vi "ProcessData(SubVI).vi"(5 "Queue":refnum<queue>) -> ()   [LabVIEW 2013, in "main.lvlib"]
uses:
  main.lvlib
  Controls/Enum Variables.ctl
  Controls/Enum User Events.ctl
  Controls/Enum Globals.ctl
  Controls/Enum Process Data.ctl
  CreatePDF.vi
panel:
  out "Blue":dbl[][](graph)
  out "Blue index":dbl format="%d%%"
  in  "ResetBlueBtn":bool
  in  "ZoomBlueBtn":bool
  out "Blue Pressure":dbl
  out "Red":dbl[][](graph)
  out "Armpressure":dbl
  in  "System Stop Button":bool
  in  "GraphSelection(Red:F)":bool
  in  "Cursor Mode":bool
  in  "ResetFrontImage":bool
  out "Red index":dbl format="%d%%"
  out "Red Pressure":dbl
  in  "ResetRedBtn":bool
  in  "ZoomRedBtn":bool
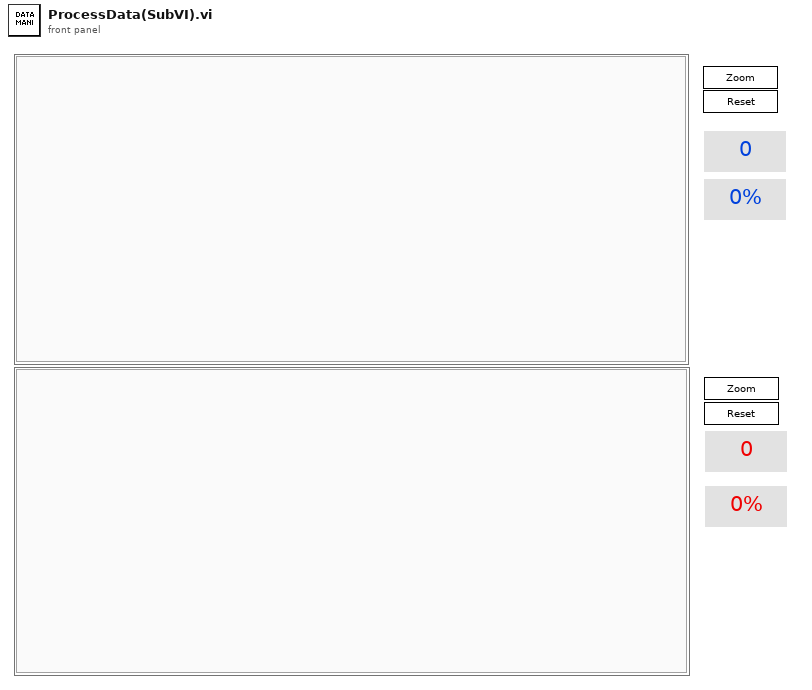
[diagram p1: front panel]
types:
  T1 = typedef "main.lvlib/Enum Process Data.ctl" = enum16{"Init", "Set Cursor Mode", "Set Data Path", "Get All"}
  T2 = typedef "main.lvlib/Enum Variables.ctl" = enum16{"SetAcqFilter", "GetAcqFilter", "Set Filter", "Get Filter", "Set Height", "Get Height", "Set Recorded Height", "Get Recorded Height", "Set Blue Pressure", "Get Blue Pressure", "Set Red Pressure", "Get Red Pressure", "Init", "Reset Pressure", "Set Red Cursors", "Get Red Cursors", "Set Blue Cursors", "Get Blue Cursors", "Set Language", "Get Language", "Set Active Graphs", "Get ActiveGraphs", "Set Method", "Get Method", "Set Encryption", "Get Encryption", "Set ExcelVersion", "Get ExcelVersion", "Set DICOM Avail", "Get DICOM Avail", "Set DICOM Encode", "Get DICOM Encode", "Set JournalExport", "Get JournalExport", "Set Sequence", "Get Sequence", "Set DAQ Connected", "Get DAQ Connected", "Set Current Graph", "Get Current Graph", "Set General Settings", "Get Hyphenation", "Set Arm Calc Method", "Get Arm Calc Method", "Set Dicom Tags", "Get Dicom Tags", "Set BT Serial", "Get BT Serial", "Set BT Accepted Serials", "Get BT Accepted Serials", "Get BT License", "Set BT License"}
  T3 = typedef "main.lvlib/Enum User Events.ctl" = enum16{"User Event", "Init"}
  T4 = typedef "main.lvlib/Enum Globals.ctl" = enum16{"Init", "Set DataPath", "Set Freq", "Get"}
  T5 = typedef "LVPoint32TypeDef.ctl" = cluster{"Horizontal":i32, "Vertical":i32}
  T6 = typedef "LVCursorListTypeDef.ctl" = cluster{"Name":string, "Color":u32, "Style":u8, "Point Style":u8, "Name Visible":bool, "Allow Drag":bool, "Cursor Mode":u32, "Plot":i32, "Index":i32, "Position":cluster{"X":dbl, "Y":dbl}, "X Scale":u32, "Y Scale":u32, "Watch Plots":i32[], "Watch All Plots":bool, "Plot Area":i32, "Label Offset":cluster{"X":dbl, "Y":dbl}}[]
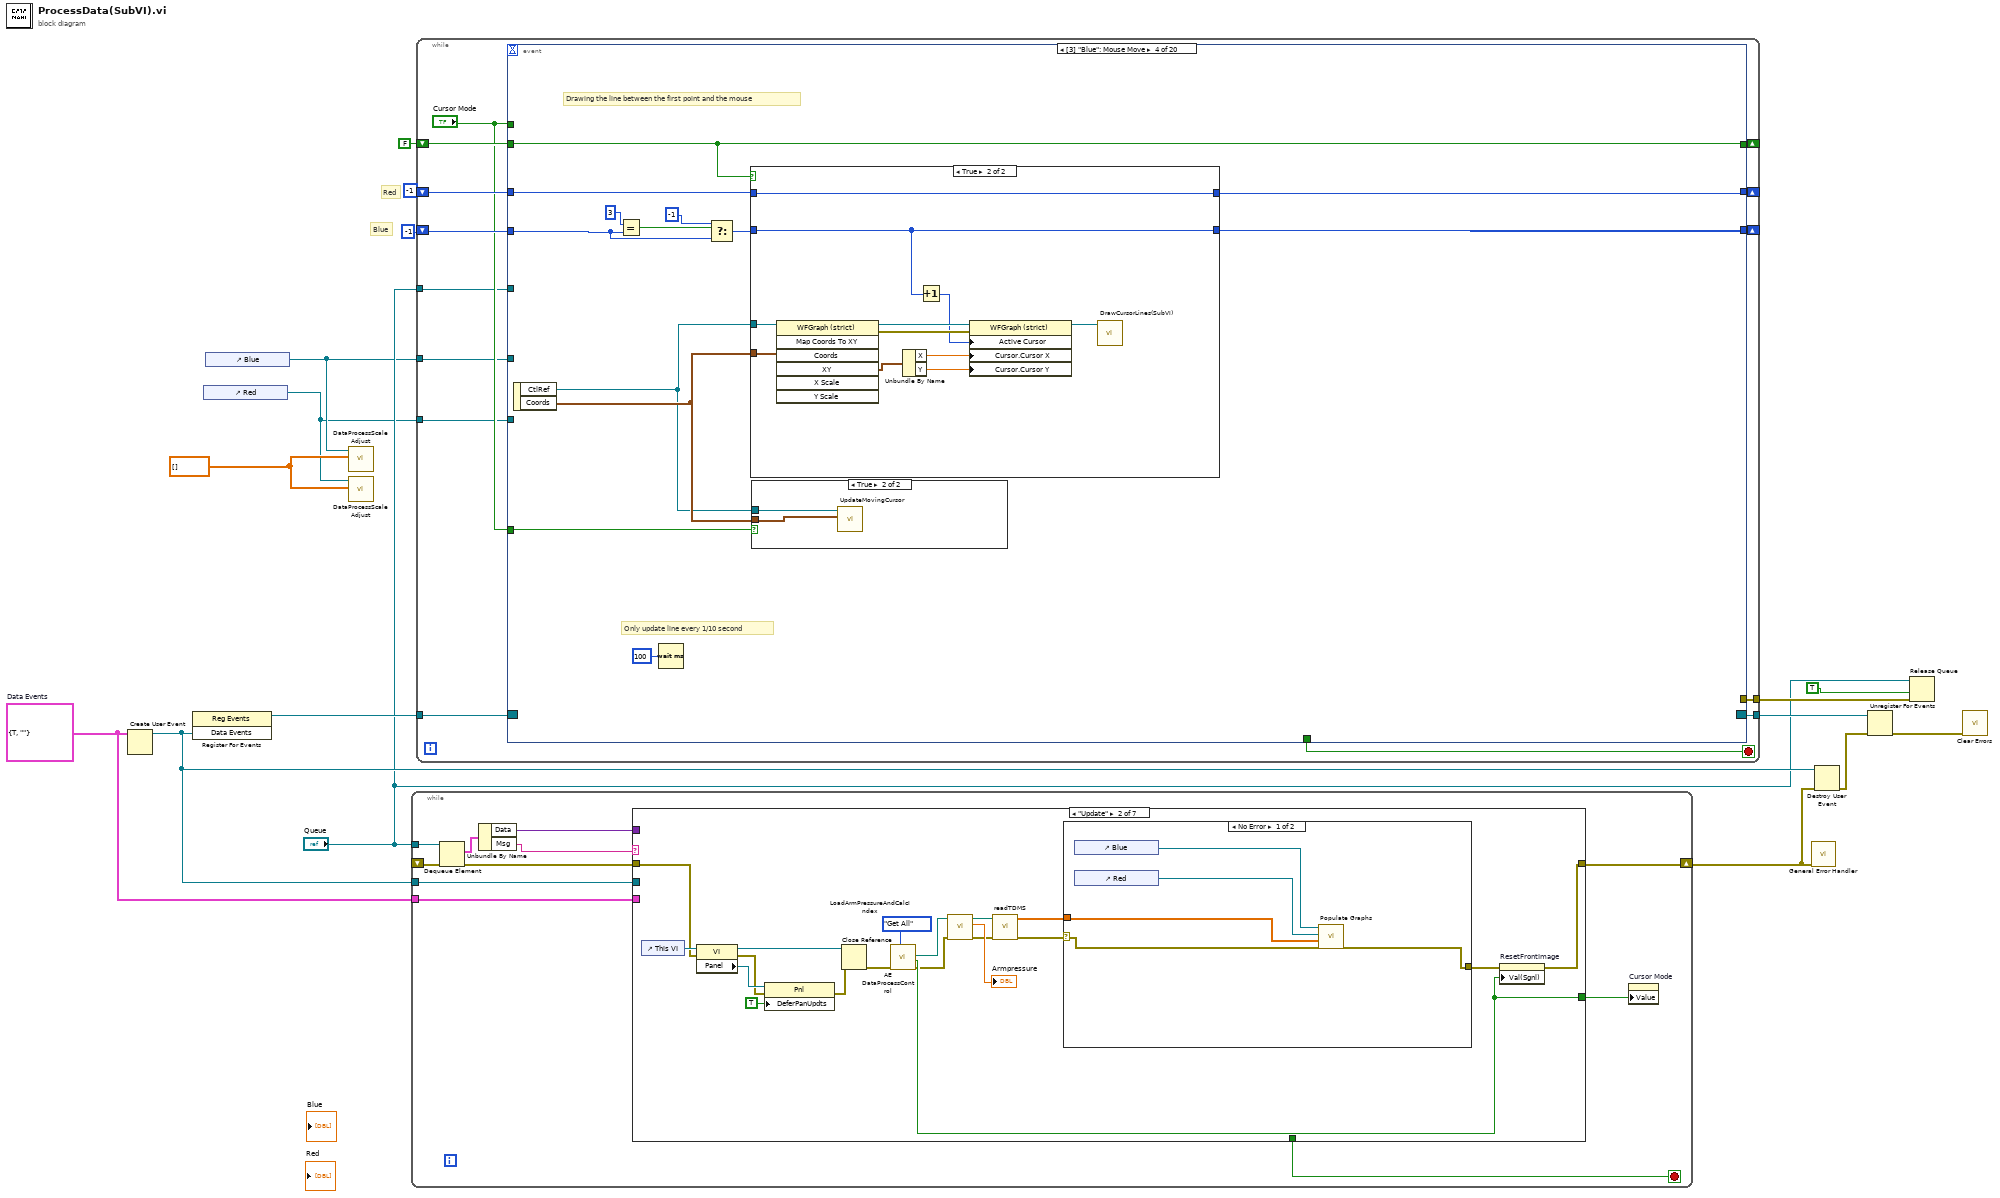
[diagram p0: block diagram]
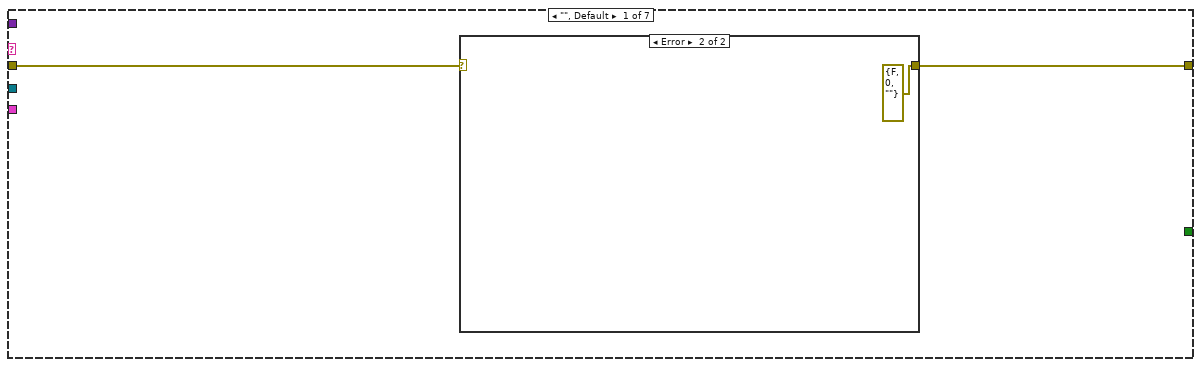
[diagram p2: hidden frame]
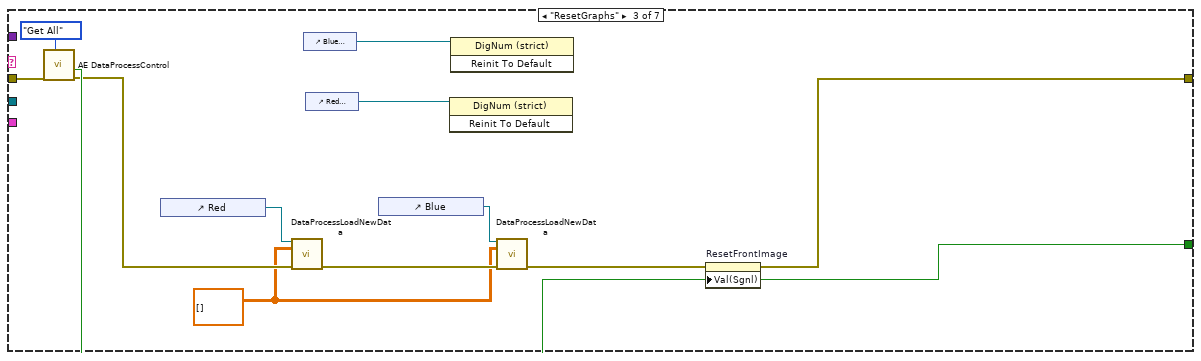
[diagram p5: hidden frame]
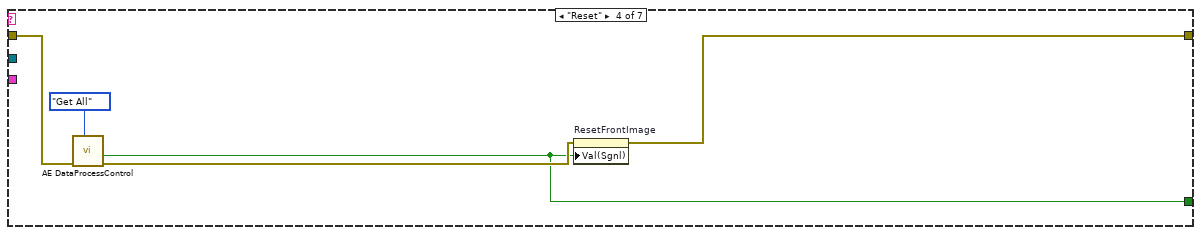
[diagram p6: hidden frame]
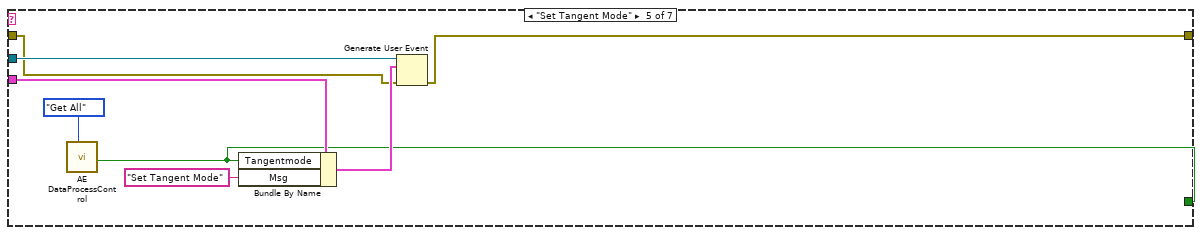
[diagram p7: hidden frame]
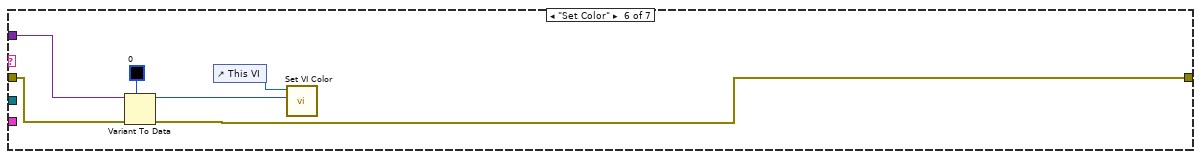
[diagram p8: hidden frame]
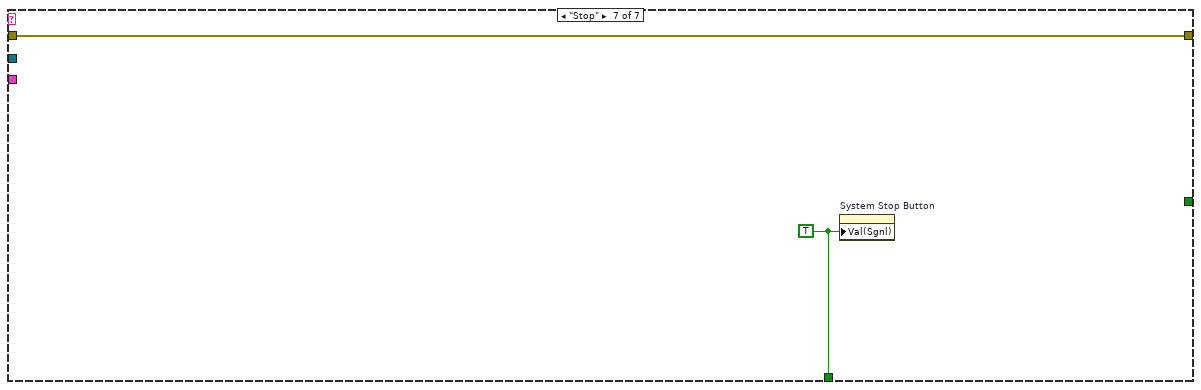
[diagram p9: hidden frame]
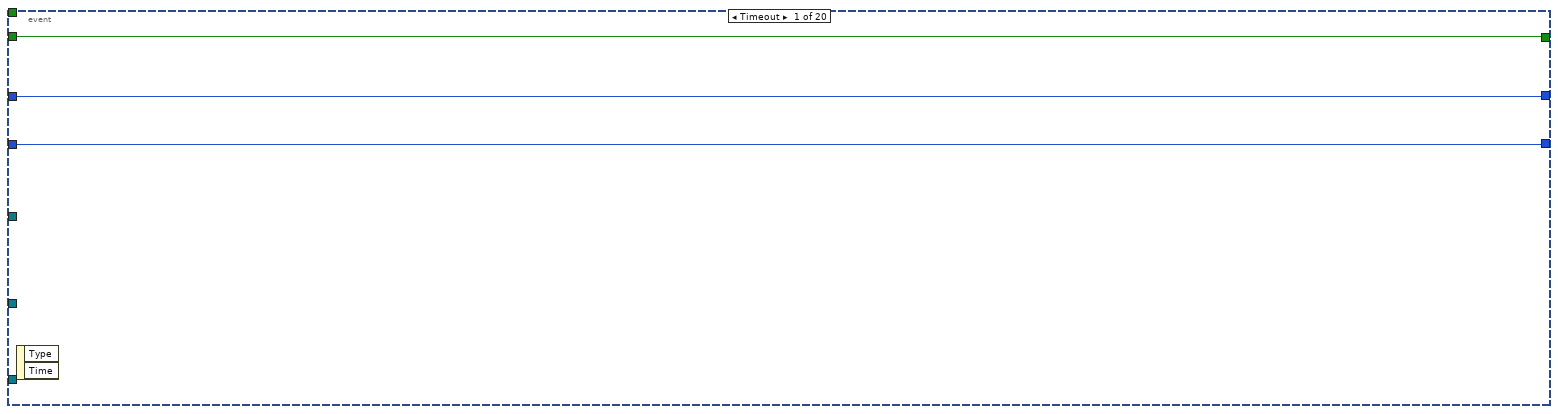
[diagram p10: hidden frame]
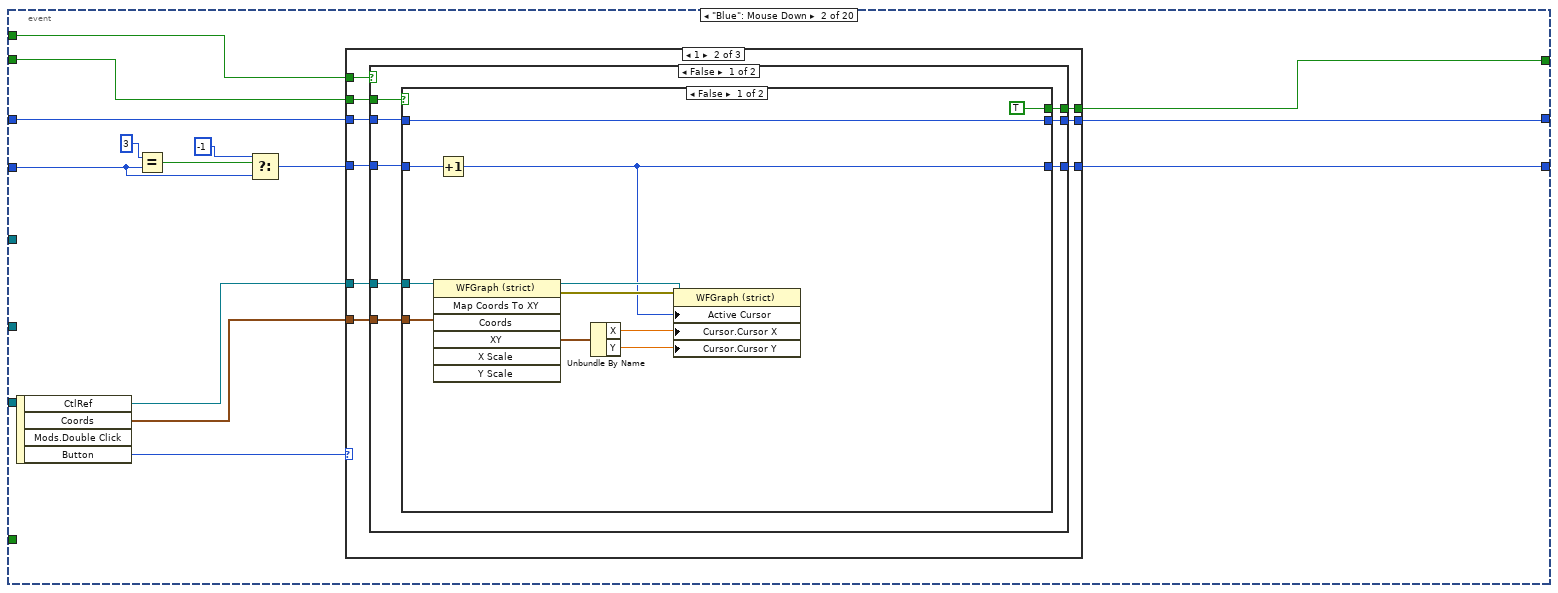
[diagram p11: hidden frame]
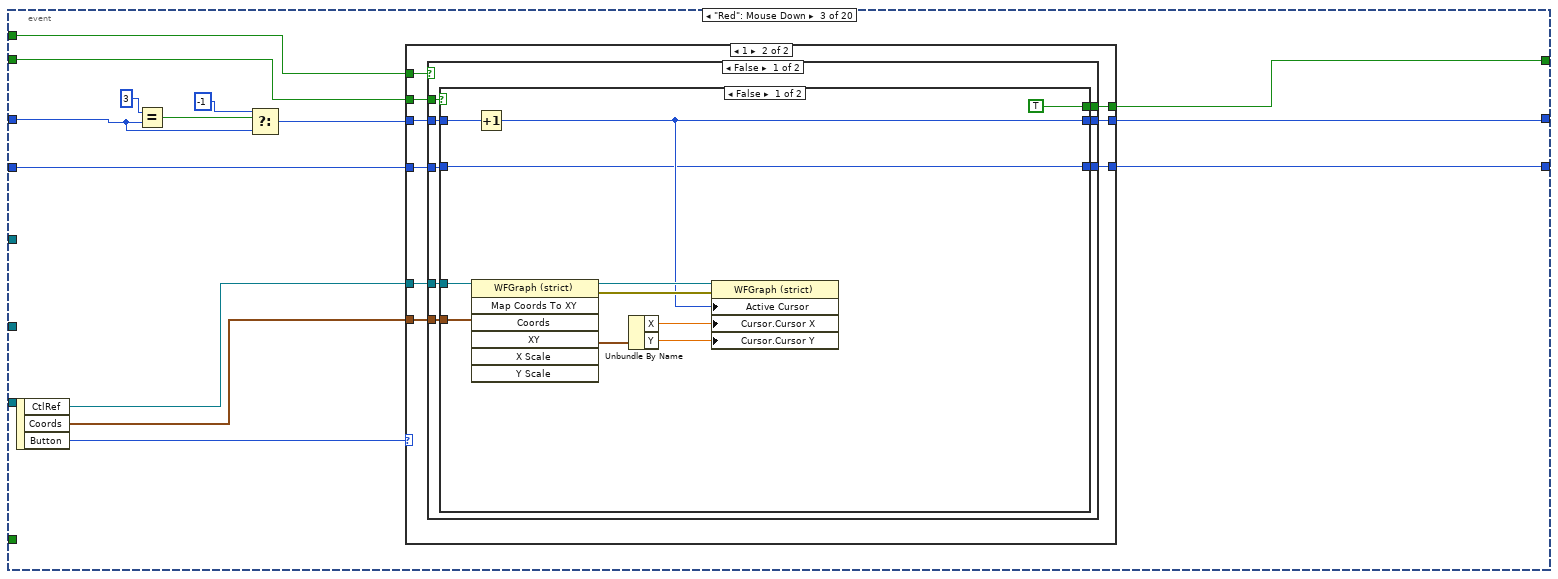
[diagram p16: hidden frame]
diagram:
  w3 = dbl[] []
  w10 = cluster{"Tangentmode":bool, "Msg":string} {"Tangentmode"=TRUE, "Msg"=""}  # Data Events
  # "Blue"
  # "Red"
  n1 = Create User Event(user event datatype=w10) -> (user event=w6:refnum<user-event>)  [unwired: 1 in, 1 out]
  n2 = register-events(w6) -> (reference out=w11:refnum<event-registration>)  [unwired: 2 in, 1 out]
  n3 = control-ref of="Red"() -> (w1:refnum<vi>)
  n4 = control-ref of="Blue"() -> (w2:refnum<vi>)
  n5 = call "DataProcessScaleAdjust.vi"(10:"Graph"=w3, 11:"Graph"=w2) -> ()  [unwired: 8 in, 2 out]
  n6 = call "DataProcessScaleAdjust.vi"(10:"Graph"=w3, 11:"Graph"=w1) -> ()  [unwired: 8 in, 2 out]
  n7 = while {
    tunnel: "Queue" -> [w26]
    shift-right: [w25] -> w7
    shift-left: _ -> [w24]
    tunnel: w6 -> [w22]
    tunnel: w10 -> [w21]
    stop <- w17 stop-if-true
    n8 = Dequeue Element(queue=w26, error in (no error)=w24) -> (element=w20:cluster{"Msg":string, "Data":variant}, error out=w27:errorcluster)  [unwired: 1 in, 2 out]
    n9 = Unbundle By Name(w20) -> ("Data"=w18:variant, "Msg"=w19:string)
    n10 = case shown="\"Update\"" w19 {
      tunnel: w27 -> [w29 w34 w62 w71 w75 w83 w89]
      tunnel: [w28 w36 w64 w73 w74 w82 w89] -> w25
      tunnel: [_ w43 w61 w69 w76 _ _] -> w23
      tunnel: [_ _ _ _ _ _ w88] -> w17
      tunnel: w22 -> [_ _ _ _ w81 _ _]
      tunnel: w21 -> [_ _ _ _ w79 _ _]
      tunnel: w18 -> [_ _ _ _ _ w86 _]
      frame "", Default {
        n11 = case shown="Error" w29 {
          selector: w29 -> [w30 _]
          tunnel: [w30 errorcluster {"status"=FALSE, "code"=0, "source"=""} ("error IO")] -> w28
          frame No Error {
          }
          frame Error {
          }
        }
      }
      frame "Update" {
        n12 = control-ref of="This VI"() -> (w41:refnum<vi>)
        n13 = property class="VI"(reference=w41, error in=w34) -> (reference out=w42:refnum<vi>, error out=w38:errorcluster, "Panel"=w40:refnum<vi>)
        n14 = property class="Pnl"(reference=w40, error in=w38, "DeferPanUpdts"=TRUE ("Defer Panel Updates")) -> (error out=w39:errorcluster)  [unwired: 1 out]
        n15 = Close Reference(reference=w42, error in (no error)=w39) -> (error out=w32:errorcluster)
        n16 = call "AE DataProcessControl.vi"("Action"=Enum_Process_Data."Get All", "error in (no error)"=w32) -> ("error out"=w35:errorcluster, "Cursor Mode Out"=w43:bool, "Data Path Out"=w45:path)  [unwired: 7 in]
        n17 = call "LoadArmPressureAndCalcIndex.vi"("error in (no error)"=w35, "Path"=w45) -> ("error out"=w33:errorcluster, "Armpressure"=→"Armpressure":dbl, "Path Out"=w46:path)  [unwired: 7 in]
        n18 = call "readTDMS.vi"("error in (no error)"=w33, "Path Out"=w46) -> ("error out"=w49:errorcluster, "Array"=w50:dbl[][])  [unwired: 8 in]
        n19 = case shown="No Error" w49 {
          selector: w49 -> [w51 w56]
          tunnel: w50 -> [w53 _]
          tunnel: [w55 w56] -> w48
          frame No Error {
            n20 = control-ref of="Blue"() -> (w54:refnum<vi>)
            n21 = control-ref of="Red"() -> (w52:refnum<vi>)
            n22 = call "Populate Graphs.vi"("error in (no error)"=w51, "Array"=w53, "Red"=w52, "Blue"=w54) -> ("error out"=w55:errorcluster)  [unwired: 7 in]
          }
          frame Error {
          }
        }
        n23 = property on="ResetFrontImage" class="Bool (strict)"(error in=w48, "Val(Sgnl)"=w43) -> (error out=w36:errorcluster)  [unwired: 1 in, 1 out]
      }
      frame "ResetGraphs" {
        w58 = dbl[][] [] ("Data Blue")
        n24 = call "AE DataProcessControl.vi"("Action"=Enum_Process_Data."Get All", "error in (no error)"=w62) -> ("error out"=w59:errorcluster, "Cursor Mode Out"=w61:bool)  [unwired: 7 in, 1 out]
        n25 = control-ref of="Red"() -> (w57:refnum<vi>)
        n26 = call "DataProcessLoadNewData.vi"("Graph"=w57, "Data"=w58, "error in (no error)"=w59) -> ("error out"=w60:errorcluster)  [unwired: 11 in, 1 out]
        n27 = control-ref of="Blue Pressure"() -> (w66:refnum<vi>)
        n28 = control-ref of="Red Pressure"() -> (w65:refnum<vi>)
        n29 = control-ref of="Blue"() -> (w67:refnum<vi>)
        n30 = invoke class="DigNum (strict)" method="Reinit To Default"(reference=w65) -> ()  [unwired: 2 in, 3 out]
        n31 = invoke class="DigNum (strict)" method="Reinit To Default"(reference=w66) -> ()  [unwired: 2 in, 3 out]
        n32 = call "DataProcessLoadNewData.vi"("Graph"=w67, "Data"=w58, "error in (no error)"=w60) -> ("error out"=w68:errorcluster)  [unwired: 11 in, 1 out]
        n33 = property on="ResetFrontImage" class="Bool (strict)"(error in=w68, "Val(Sgnl)"=w61) -> (error out=w64:errorcluster)  [unwired: 1 in, 1 out]
      }
      frame "Reset" {
        n34 = call "AE DataProcessControl.vi"("Action"=Enum_Process_Data."Get All", "error in (no error)"=w71) -> ("error out"=w70:errorcluster, "Cursor Mode Out"=w69:bool)  [unwired: 7 in, 1 out]
        n35 = property on="ResetFrontImage" class="Bool (strict)"(error in=w70, "Val(Sgnl)"=w69) -> (error out=w73:errorcluster)  [unwired: 1 in, 1 out]
      }
      frame "Set Tangent Mode" {
        n36 = call "AE DataProcessControl.vi"("Action"=Enum_Process_Data."Get All") -> ("Cursor Mode Out"=w76:bool)  [unwired: 8 in, 2 out]
        n37 = Bundle By Name(cluster=w79, "Tangentmode"=w76, "Msg"="Set Tangent Mode") -> (w78:cluster{"Tangentmode":bool, "Msg":string})
        n38 = Generate User Event(user event=w81, event data cluster=w78, error in=w75) -> (error out=w74:errorcluster)  [unwired: 1 in, 1 out]
      }
      frame "Set Color" {
        n39 = Variant To Data(error in=w83, type=u32 0, Variant=w86) -> (data=w85:u32, error out=w82:errorcluster)
        n40 = control-ref of="This VI"() -> (w87:refnum<vi>)
        n41 = call "Set VI Color.vi"("Pane Color"=w85, "VI in"=w87) -> ()  [unwired: 10 in]
      }
      frame "Stop" {
        w88 = TRUE
        n42 = property on="System Stop Button" class="Bool (strict)"("Val(Sgnl)"=w88) -> ()  [unwired: 2 in, 2 out]
      }
    }
    n43 = property on="Cursor Mode" class="Bool (strict)"("Value"=w23) -> ()  [unwired: 2 in, 2 out]
  }
  n44 = while {
    shift-right: [w102] -> _
    shift-left: -1 -> [w99]
    shift-right: [w101] -> _
    shift-left: -1 -> [w100]
    shift-right: [w98] -> _
    shift-left: FALSE -> [w97]
    tunnel: w2 -> [w95]
    tunnel: w1 -> [w94]
    tunnel: "Queue" -> [w93]
    tunnel: [w92] -> w12
    tunnel: w11 -> [w91]
    tunnel: [w90] -> w9
    stop <- w103 stop-if-true
    n45 = event shown="[3] \"Blue\": Mouse Move" {
      selector: w91 -> [_ _ _ _ _ _ _ _ _ _ _ _ _ _ _ _ _ _ _ _]
      dyn-events: [_ _ _ _ _ _ _ _ _ _ _ _ _ _ _ _ _ _ _ _] -> w90
      timeout: _ -> [_ _ _ _ _ _ _ _ _ _ _ _ _ _ _ _ _ _ _ _]
      tunnel: [_ _ _ _ _ _ _ _ _ _ _ _ _ "System Stop Button" _ _ _ _ _ _] -> w103
      tunnel: [w106 w118 w172 w224 w252 w292 w380 w446 w469 w494 w521 w547 w587 w591 w596 w613 w632 w655 w673 w687] -> w102
      tunnel: [w105 w117 w171 w223 w251 w290 w378 w449 w472 w493 w520 w546 w586 w590 w597 w612 w631 w654 w674 w686] -> w101
      tunnel: w100 -> [w105 w112 w165 w216 w244 w287 w375 w450 w473 w493 w520 w546 w586 w590 w597 w612 w631 w654 w674 w686]
      tunnel: w99 -> [w106 w116 w166 w222 w246 w291 w379 w447 w470 w494 w521 w547 w587 w591 w596 w613 w632 w655 w673 w687]
      tunnel: [w104 w109 w162 w221 w250 w288 w376 w448 w471 w492 w522 w545 w588 w589 w595 w614 w633 w656 w675 w688] -> w98
      tunnel: w97 -> [w104 w110 w164 w221 w250 w289 w377 w451 w474 w492 w522 w545 w588 w589 w595 w614 w633 w656 w675 w688]
      tunnel: "Cursor Mode" -> [_ w108 w163 _ _ w286 w374 w445 w468 _ _ _ _ _ _ _ _ _ _ _]
      tunnel: "Cursor Mode" -> [_ _ _ w214 w241 _ _ _ _ _ _ _ _ _ _ _ _ _ _ _]
      tunnel: w95 -> [_ _ _ _ _ _ _ _ _ _ w496 w551 _ _ _ w610 _ _ _ _]
      tunnel: w94 -> [_ _ _ _ _ _ _ _ _ _ w495 w550 _ _ w593 _ _ _ _ _]
      tunnel: w93 -> [_ _ _ _ _ _ _ _ _ _ _ _ _ _ w594 w611 _ _ _ w690]
      tunnel: [_ _ _ _ _ w274 _ _ _ _ _ _ _ _ _ _ _ _ _ _] -> w92
      event Timeout {
        n46 = event-data() -> ()  [unwired: 1 in, 2 out]
      }
      event "Blue": Mouse Down {
        n47 = event-data() -> ("CtlRef"=w120:refnum<vi>, "Coords"=w119:T5, "Button"=w107:u16)  [unwired: 1 in, 1 out]
        n48 = Equal?(x=3, y=w112) -> (x = y?=w113:bool)
        n49 = Select(t=-1, s=w113, f=w112) -> (s? t:f=w111:i32)
        n50 = case shown="1" w107 {
          tunnel: w120 -> [_ w132 _]
          tunnel: w119 -> [_ w131 _]
          tunnel: [w123 w130 w159] -> w118
          tunnel: [w122 w129 w158] -> w117
          tunnel: w116 -> [w123 w128 w159]
          tunnel: w111 -> [w122 w127 w158]
          tunnel: w110 -> [w121 w126 w160]
          tunnel: [w121 w125 w160] -> w109
          tunnel: w108 -> [_ w124 _]
          frame 0, Default {
          }
          frame 1 {
            n51 = case shown="False" w124 {
              tunnel: w132 -> [w140 _]
              tunnel: w131 -> [w139 _]
              tunnel: [w138 w157] -> w130
              tunnel: [w137 w156] -> w129
              tunnel: w128 -> [w136 w157]
              tunnel: w127 -> [w135 w156]
              tunnel: w126 -> [w134 w155]
              tunnel: [w133 w155] -> w125
              frame False {
                n52 = case shown="False" w134 {
                  selector: w134 -> [_ w152]
                  tunnel: w140 -> [w151 _]
                  tunnel: w139 -> [w150 _]
                  tunnel: w135 -> [w143 w154]
                  tunnel: [w142 w154] -> w137
                  tunnel: w136 -> [w144 w153]
                  tunnel: [w144 w153] -> w138
                  tunnel: [TRUE w152] -> w133
                  frame False {
                    n53 = invoke class="WFGraph (strict)" method="Map Coords To XY"(reference=w151, "Coords"=w150) -> (reference out=w149:refnum<vi>, error out=w148:errorcluster, "XY"=w147:cluster{"X":dbl, "Y":dbl})  [unwired: 5 in, 4 out]
                    n54 = Increment(x=w143) -> (x+1=w142:i32)
                    n55 = Unbundle By Name(w147) -> ("X"=w146:dbl, "Y"=w145:dbl)
                    n56 = property class="WFGraph (strict)"(reference=w149, error in=w148, "Active Cursor"=w142, "Cursor.Cursor X"=w146, "Cursor.Cursor Y"=w145) -> ()  [unwired: 2 out]
                  }
                  frame True {
                  }
                }
              }
              frame True {
              }
            }
          }
          frame 2 {
          }
        }
      }
      event "Red": Mouse Down {
        n57 = event-data() -> ("CtlRef"=w174:refnum<vi>, "Coords"=w173:T5, "Button"=w161:u16)  [unwired: 1 in]
        n58 = Equal?(x=3, y=w166) -> (x = y?=w168:bool)
        n59 = Select(t=-1, s=w168, f=w166) -> (s? t:f=w167:i32)
        n60 = case shown="1" w161 {
          tunnel: w174 -> [_ w186]
          tunnel: w173 -> [_ w185]
          tunnel: [w176 w184] -> w172
          tunnel: [w175 w183] -> w171
          tunnel: w167 -> [w176 w182]
          tunnel: w165 -> [w175 w181]
          tunnel: w164 -> [w177 w180]
          tunnel: w163 -> [_ w179]
          tunnel: [w177 w178] -> w162
          frame 0, Default {
          }
          frame 1 {
            n61 = case shown="False" w179 {
              tunnel: w186 -> [w194 _]
              tunnel: w185 -> [w193 _]
              tunnel: [w192 w211] -> w184
              tunnel: [w191 w209] -> w183
              tunnel: w182 -> [w190 w211]
              tunnel: w181 -> [w189 w209]
              tunnel: w180 -> [w188 w210]
              tunnel: [w187 w210] -> w178
              frame False {
                n62 = case shown="False" w188 {
                  selector: w188 -> [_ w206]
                  tunnel: w194 -> [w205 _]
                  tunnel: w193 -> [w204 _]
                  tunnel: w189 -> [w196 w208]
                  tunnel: [w196 w208] -> w191
                  tunnel: w190 -> [w198 w207]
                  tunnel: [w197 w207] -> w192
                  tunnel: [TRUE w206] -> w187
                  frame False {
                    n63 = invoke class="WFGraph (strict)" method="Map Coords To XY"(reference=w205, "Coords"=w204) -> (reference out=w203:refnum<vi>, error out=w202:errorcluster, "XY"=w201:cluster{"X":dbl, "Y":dbl})  [unwired: 5 in, 4 out]
                    n64 = Increment(x=w198) -> (x+1=w197:i32)
                    n65 = Unbundle By Name(w201) -> ("X"=w200:dbl, "Y"=w199:dbl)
                    n66 = property class="WFGraph (strict)"(reference=w203, error in=w202, "Active Cursor"=w197, "Cursor.Cursor X"=w200, "Cursor.Cursor Y"=w199) -> ()  [unwired: 2 out]
                  }
                  frame True {
                  }
                }
              }
              frame True {
              }
            }
          }
        }
      }
      event "Blue": Mouse Move {
        # "Only update line every 1/10 second"
        # "Drawing the line between the first point and the mouse"
        n67 = event-data() -> ("CtlRef"=w213:refnum<vi>, "Coords"=w215:T5)  [unwired: 1 in]
        n68 = Equal?(x=3, y=w216) -> (x = y?=w218:bool)
        n69 = Wait (ms)(milliseconds to wait=u32 100) -> ()  [unwired: 1 out]
        n70 = Select(t=-1, s=w218, f=w216) -> (s? t:f=w217:i32)
        n71 = case shown="True" w221 {
          tunnel: w213 -> [_ w239]
          tunnel: w215 -> [_ w238]
          tunnel: w217 -> [w228 w230]
          tunnel: [w228 w230] -> w223
          tunnel: w222 -> [w227 w232]
          tunnel: [w227 w232] -> w224
          frame False {
          }
          frame True {
            n72 = invoke class="WFGraph (strict)" method="Map Coords To XY"(reference=w239, "Coords"=w238) -> (reference out=w237:refnum<vi>, error out=w236:errorcluster, "XY"=w235:cluster{"X":dbl, "Y":dbl})  [unwired: 5 in, 4 out]
            n73 = Unbundle By Name(w235) -> ("X"=w234:dbl, "Y"=w233:dbl)
            n74 = Increment(x=w230) -> (x+1=w231:i32)
            n75 = property class="WFGraph (strict)"(reference=w237, error in=w236, "Active Cursor"=w231, "Cursor.Cursor X"=w234, "Cursor.Cursor Y"=w233) -> (reference out=w229:refnum<vi>)  [unwired: 1 out]
            n76 = call "DrawCursorLines(SubVI).vi"("CtlRef"=w229) -> ()  [unwired: 9 in, 2 out]
          }
        }
        n77 = case shown="True" w214 {
          tunnel: w213 -> [_ w225]
          tunnel: w215 -> [_ w226]
          frame False {
          }
          frame True {
            n78 = call "UpdateMovingCursor.vi"("Coords"=w226, "CtlRef"=w225) -> ()  [unwired: 8 in]
          }
        }
      }
      event "Red": Mouse Move {
        # "Only update line every 1/10 second"
        n79 = event-data() -> ("CtlRef"=w243:refnum<vi>, "Coords"=w242:T5)  [unwired: 1 in]
        n80 = Wait (ms)(milliseconds to wait=u32 100) -> ()  [unwired: 1 out]
        n81 = Equal?(x=3, y=w246) -> (x = y?=w247:bool)
        n82 = Select(t=-1, s=w247, f=w246) -> (s? t:f=w245:i32)
        n83 = case shown="True" w241 {
          tunnel: w243 -> [w254 _]
          tunnel: w242 -> [w253 _]
          frame True {
            n84 = call "UpdateMovingCursor.vi"("Coords"=w253, "CtlRef"=w254) -> ()  [unwired: 8 in]
          }
          frame False {
          }
        }
        n85 = case shown="True" w250 {
          tunnel: w243 -> [_ w267]
          tunnel: w242 -> [_ w266]
          tunnel: w244 -> [w256 w259]
          tunnel: [w256 w259] -> w251
          tunnel: w245 -> [w255 w258]
          tunnel: [w255 w258] -> w252
          frame False {
          }
          frame True {
            n86 = invoke class="WFGraph (strict)" method="Map Coords To XY"(reference=w267, "Coords"=w266) -> (reference out=w265:refnum<vi>, error out=w264:errorcluster, "XY"=w263:cluster{"X":dbl, "Y":dbl})  [unwired: 5 in, 4 out]
            n87 = Unbundle By Name(w263) -> ("X"=w262:dbl, "Y"=w261:dbl)
            n88 = Increment(x=w258) -> (x+1=w260:i32)
            n89 = property class="WFGraph (strict)"(reference=w265, error in=w264, "Active Cursor"=w260, "Cursor.Cursor X"=w262, "Cursor.Cursor Y"=w261) -> (reference out=w257:refnum<vi>)  [unwired: 1 out]
            n90 = call "DrawCursorLines(SubVI).vi"("CtlRef"=w257) -> ()  [unwired: 9 in, 2 out]
          }
        }
      }
      event "Blue": Mouse Up {
        n91 = event-data() -> ("CtlRef"=w283:refnum<vi>, "Coords"=w284:T5, "Button"=w285:u16)  [unwired: 1 in, 1 out]
        n92 = case shown="1" w285 {
          tunnel: [w295 w308] -> w292
          tunnel: w291 -> [w295 w307]
          tunnel: [w294 w306] -> w290
          tunnel: w289 -> [w293 w305]
          tunnel: [w293 w304] -> w288
          tunnel: w287 -> [w294 w303]
          tunnel: w286 -> [_ w302]
          tunnel: w283 -> [_ w301]
          tunnel: w284 -> [_ w300]
          tunnel: [_ w299] -> w279
          tunnel: w284 -> [_ w298]
          tunnel: w283 -> [_ w297]
          tunnel: [_ w296] -> w282
          frame 0, Default {
          }
          frame 1 {
            n93 = case shown="True" w302 {
              tunnel: w300 -> [w319 _]
              tunnel: [w318 w354] -> w308
              tunnel: w307 -> [w317 w354]
              tunnel: [w316 w353] -> w306
              tunnel: w301 -> [w315 _]
              tunnel: w305 -> [w314 w355]
              tunnel: [w313 w355] -> w304
              tunnel: w303 -> [w312 w353]
              tunnel: w297 -> [w311 w352]
              tunnel: [w310 w350] -> w299
              tunnel: w298 -> [_ w351]
              tunnel: [w309 _] -> w296
              frame False {
                n94 = case shown="True" w314 {
                  selector: w314 -> [w321 _]
                  tunnel: w315 -> [_ _]
                  tunnel: w319 -> [_ _]
                  tunnel: w312 -> [w323 w343]
                  tunnel: [w323 w342] -> w316
                  tunnel: w317 -> [w322 w344]
                  tunnel: [w322 w344] -> w318
                  tunnel: [w321 FALSE] -> w313
                  tunnel: w311 -> [_ w333]
                  tunnel: [0.0 w328] -> w310
                  tunnel: [_ w330] -> w309
                  frame False {
                  }
                  frame True {
                    n95 = property class="WFGraph (strict)"(reference=w333) -> (reference out=w329:refnum<vi>, "CrsrList"=w327:T6)  [unwired: 1 in, 1 out]
                    n96 = Increment(x=w343) -> (x+1=w342:i32)
                    n97 = call "AE Acquisition.vi"("Action"=Enum_Globals."Get") -> ("Freq Out"=w325:i32)  [unwired: 7 in, 3 out]
                    n98 = call "CalcXValue(SubVI).vi"("CrsrList"=w327) -> ("X-value"=w326:dbl)  [unwired: 8 in, 2 out]
                    n99 = Multiply(x=w325, y=w326) -> (x*y=w337:dbl)
                    n100 = property class="WFGraph (strict)"(reference=w329) -> ("Value"=w324:dbl[][])  [unwired: 1 in, 2 out]
                    n101 = Greater?(x=w337, y=0.0) -> (0:w335:bool)
                    n102 = call "DrawCursorLines(SubVI).vi"("CtlRef"=w329) -> ("Array"=w331:dbl[][], "reference out"=w332:refnum<vi>)  [unwired: 9 in]
                    n103 = Index Array(array=w324, index (row)=1) -> (element=w339:dbl[])  [unwired: 1 in]
                    n104 = case shown="True" w335 {
                      tunnel: w339 -> [_ w349]
                      tunnel: w337 -> [_ w348]
                      tunnel: [0.0 w346] -> w340
                      frame False {
                      }
                      frame True {
                        n105 = Index Array(array=w349, index=w348) -> (element=w347:dbl)
                        n106 = Decrement(x=w347) -> (x-1=w346:dbl)
                      }
                    }
                    n107 = Round To Nearest(number=w340) -> (nearest integer value=w328:dbl)
                    n108 = call "PlotPressureAtGraph.vi"("Press In"=w328, "Array"=w331, "reference"=w332) -> ("Array Out"=w330:dbl[][])  [unwired: 8 in]
                  }
                }
              }
              frame True {
                n109 = call "GetPressureAtMouse.vi"("Coords"=w351, "GraphRefnum"=w352) -> ("Numeric"=w350:dbl)  [unwired: 1 out]
              }
            }
          }
        }
        "Blue Pressure" <- w279
        n110 = property on="Armpressure" class="DigNum (strict)"() -> ("Value"=w275:dbl)  [unwired: 2 in, 2 out]
        n111 = Divide(x=w279, y=w275) -> (x/y=w281:dbl)
        n112 = Multiply(x=w281, y=100.0) -> (x*y=w277:dbl)
        n113 = Less Or Equal To 0?(x=w275) -> (x <= 0?=w276:bool)
        n114 = Select(t=w275, s=w276, f=w277) -> (s? t:f=→"Blue index":dbl)
        n115 = call "AE Variables.vi"("VariantIn"=w282, "Action"=Enum_Variables."Set Blue Cursors") -> ("error out"=w270:errorcluster)  [unwired: 10 in, 7 out]
        n116 = call "AE Variables.vi"("VariantIn"=w279, "error in (no error)"=w270, "Action"=Enum_Variables."Set Blue Pressure") -> ("error out"=w268:errorcluster)  [unwired: 9 in, 7 out]
        n117 = call "AE User Events.vi"("Action"=Enum_User_Events."User Event", "error in (no error)"=w268, "User Event"="SavePressure") -> ("error out"=w274:errorcluster)  [unwired: 7 in, 1 out]
      }
      event "Red": Mouse Up {
        n118 = event-data() -> ("CtlRef"=w371:refnum<vi>, "Coords"=w372:T5, "Button"=w373:u16)  [unwired: 1 in, 1 out]
        n119 = case shown="1" w373 {
          tunnel: [w383 w396] -> w380
          tunnel: w379 -> [w383 w395]
          tunnel: [w382 w394] -> w378
          tunnel: w377 -> [w381 w393]
          tunnel: [w381 w392] -> w376
          tunnel: w375 -> [w382 w391]
          tunnel: w374 -> [_ w390]
          tunnel: w371 -> [_ w389]
          tunnel: w372 -> [_ w388]
          tunnel: [_ w387] -> w369
          tunnel: w372 -> [_ w386]
          tunnel: w371 -> [_ w385]
          tunnel: [_ w384] -> w370
          frame 0, Default {
          }
          frame 1 {
            n120 = case shown="True" w390 {
              tunnel: w388 -> [w407 _]
              tunnel: [w398 w443] -> w396
              tunnel: w395 -> [w406 w443]
              tunnel: [w405 w442] -> w394
              tunnel: w389 -> [w404 _]
              tunnel: w393 -> [w403 w444]
              tunnel: [w402 w444] -> w392
              tunnel: w391 -> [w401 w442]
              tunnel: w385 -> [w400 w441]
              tunnel: [w399 w439] -> w387
              tunnel: w386 -> [_ w440]
              tunnel: [w397 _] -> w384
              frame False {
                n121 = case shown="True" w403 {
                  selector: w403 -> [w409 _]
                  tunnel: w404 -> [_ _]
                  tunnel: w407 -> [_ _]
                  tunnel: w401 -> [w411 w423]
                  tunnel: [w411 w423] -> w405
                  tunnel: w406 -> [w410 w422]
                  tunnel: [w410 w421] -> w398
                  tunnel: [w409 FALSE] -> w402
                  tunnel: w400 -> [_ w420]
                  tunnel: [0.0 w413] -> w399
                  tunnel: [_ w415] -> w397
                  frame False {
                  }
                  frame True {
                    # "Tryk"
                    n122 = property class="WFGraph (strict)"(reference=w420) -> (reference out=w419:refnum<vi>, "CrsrList"=w426:T6)  [unwired: 1 in, 1 out]
                    n123 = Increment(x=w422) -> (x+1=w421:i32)
                    n124 = call "AE Acquisition.vi"("Action"=Enum_Globals."Get") -> ("Freq Out"=w424:i32)  [unwired: 7 in, 3 out]
                    n125 = call "CalcXValue(SubVI).vi"("CrsrList"=w426) -> ("X-value"=w412:dbl)  [unwired: 8 in, 2 out]
                    n126 = Multiply(x=w424, y=w412) -> (x*y=w414:dbl)
                    n127 = property class="WFGraph (strict)"(reference=w419) -> (reference out=w418:refnum<vi>, "Value"=w429:dbl[][])  [unwired: 1 in, 1 out]
                    n128 = Greater?(x=w414, y=0.0) -> (0:w427:bool)
                    n129 = call "DrawCursorLines(SubVI).vi"("CtlRef"=w418) -> ("Array"=w416:dbl[][], "reference out"=w417:refnum<vi>)  [unwired: 9 in]
                    n130 = Index Array(array=w429, index (row)=1) -> (element=w431:dbl[])  [unwired: 1 in]
                    n131 = case shown="True" w427 {
                      tunnel: w431 -> [_ w438]
                      tunnel: w414 -> [_ w437]
                      tunnel: [0.0 w436] -> w432
                      frame False {
                      }
                      frame True {
                        n132 = Index Array(array=w438, index=w437) -> (element=w435:dbl)
                        n133 = Decrement(x=w435) -> (x-1=w436:dbl)
                      }
                    }
                    n134 = Round To Nearest(number=w432) -> (nearest integer value=w413:dbl)
                    n135 = call "PlotPressureAtGraph.vi"("Press In"=w413, "Array"=w416, "reference"=w417) -> ("Array Out"=w415:dbl[][])  [unwired: 8 in]
                  }
                }
              }
              frame True {
                n136 = call "GetPressureAtMouse.vi"("Coords"=w440, "GraphRefnum"=w441) -> ("Numeric"=w439:dbl)  [unwired: 1 out]
              }
            }
          }
        }
        "Red Pressure" <- w369
        n137 = property on="Armpressure" class="DigNum (strict)"() -> ("Value"=w363:dbl)  [unwired: 2 in, 2 out]
        n138 = Divide(x=w369, y=w363) -> (x/y=w368:dbl)
        n139 = Multiply(x=w368, y=100.0) -> (x*y=w364:dbl)
        n140 = Less Or Equal To 0?(x=w363) -> (x <= 0?=w366:bool)
        n141 = Select(t=w363, s=w366, f=w364) -> (s? t:f=→"Red index":dbl)
        n142 = call "AE Variables.vi"("VariantIn"=w370, "Action"=Enum_Variables."Set Red Cursors") -> ("error out"=w358:errorcluster)  [unwired: 10 in, 7 out]
        n143 = To Variant(anything=w369) -> (Variant=w359:variant)
        n144 = call "AE Variables.vi"("VariantIn"=w359, "error in (no error)"=w358, "Action"=Enum_Variables."Set Red Pressure") -> ("error out"=w356:errorcluster)  [unwired: 9 in, 7 out]
        n145 = call "AE User Events.vi"("Action"=Enum_User_Events."User Event", "error in (no error)"=w356, "User Event"="SavePressure") -> ()  [unwired: 7 in, 2 out]
      }
      event "Blue": Mouse Leave {
        n146 = event-data() -> ()  [unwired: 1 in, 1 out]
        n147 = case shown="False" w445 {
          tunnel: w451 -> [w457 w467]
          tunnel: w450 -> [w456 w465]
          tunnel: [w455 w465] -> w449
          tunnel: [w454 w467] -> w448
          tunnel: w447 -> [w453 w466]
          tunnel: [w452 w466] -> w446
          frame False {
            n148 = case shown="False" w457 {
              selector: w457 -> [w459 _]
              tunnel: w456 -> [w460 w464]
              tunnel: [w460 w463] -> w455
              tunnel: [w459 FALSE] -> w454
              tunnel: w453 -> [w458 w461]
              tunnel: [w458 w461] -> w452
              frame False {
              }
              frame True {
                n149 = Increment(x=w464) -> (x+1=w463:i32)
              }
            }
          }
          frame True {
          }
        }
      }
      event "Red": Mouse Leave {
        n150 = event-data() -> ()  [unwired: 1 in, 1 out]
        n151 = case shown="False" w468 {
          tunnel: w474 -> [w480 w490]
          tunnel: w473 -> [w479 w488]
          tunnel: [w478 w488] -> w472
          tunnel: [w477 w490] -> w471
          tunnel: w470 -> [w476 w489]
          tunnel: [w475 w489] -> w469
          frame False {
            n152 = case shown="False" w480 {
              selector: w480 -> [w482 _]
              tunnel: w479 -> [w483 w486]
              tunnel: [w483 w486] -> w478
              tunnel: [w482 FALSE] -> w477
              tunnel: w476 -> [w481 w485]
              tunnel: [w481 w484] -> w475
              frame False {
              }
              frame True {
                n153 = Increment(x=w485) -> (x+1=w484:i32)
              }
            }
          }
          frame True {
          }
        }
      }
      event "Blue": event type 3.0.x80000027 {
        n154 = event-data() -> ()  [unwired: 1 in, 8 out]
        n155 = event-data("Discard?"=TRUE) -> ()  [unwired: 1 in, 1 out]
      }
      event "ResetFrontImage": Value Change {
        n156 = event-data() -> ()  [unwired: 1 in, 1 out]
        n157 = Build Array(w496, w495) -> (w516:refnum<vi>[])
        n158 = for {
          tunnel: picture data[5B] ("Plot Images:Front") -> [w532]
          tunnel: w516 -> [w531] mode=indexing
          tunnel: [w524] -> w511
          tunnel: [w525] -> w515 mode=indexing
          tunnel: [w523] -> w512
          tunnel: "ResetFrontImage" -> [w528]
          n159 = property class="WFGraph (strict)"(reference=w531, "PlotImages.Front"=w532) -> (reference out=w533:refnum<vi>, error out=w530:errorcluster)  [unwired: 1 in]
          n160 = call "SetCursorNamePosition(SubVI).vi"("Graph"=w533) -> ("Graph Out"=w535:refnum<vi>)
          n161 = call "SetCursorMode.vi"("Visible"=w528, "Graph Refnum"=w535) -> ("Graph Refnum 2"=w534:refnum<vi>)  [unwired: 9 in]
          n162 = call "SetCursorNamePosition(SubVI).vi"("Graph"=w534) -> ("Graph Out"=w529:refnum<vi>)
          n163 = case shown="False" w528 {
            selector: w528 -> [w536 w542]
            tunnel: w530 -> [w540 w544]
            tunnel: [w539 w544] -> w527
            tunnel: w529 -> [w538 w543]
            tunnel: [w537 w543] -> w526
            tunnel: [w536 w542] -> w523
            frame False {
              n164 = property class="WFGraph (strict)"(reference=w538, error in=w540, "ActPaletteTool"=0 ("Palette:Active Tool")) -> (reference out=w537:refnum<vi>, error out=w539:errorcluster)
            }
            frame True {
            }
          }
          n165 = call "Hide Dynamic Tangent.vi"("error in (no error)"=w527, "Residuals"=w523, "WaveformGraph in"=w526) -> ("error out"=w524:errorcluster, "WaveformGraph out"=w525:refnum<vi>)  [unwired: 7 in]
        }
        n166 = Index Array(array=w515) -> (element #1=w514:refnum<vi>, element #2=w513:refnum<vi>)  [unwired: 2 in]
        n167 = call "LoadPressureAndTangents.vi"("error in (no error)"=w511, "Red Graph"=w513, "ResetFrontImage"=w512, "Blue Graph"=w514) -> ("error out"=w510:errorcluster, "output cluster"=w501:cluster{dbl, dbl, dbl, dbl})  [unwired: 2 in]
        n168 = control-ref of="Blue Pressure"() -> (w519:refnum<vi>)
        n169 = control-ref of="Red Pressure"() -> (w518:refnum<vi>)
        n170 = Unbundle(w501) -> (w500:dbl, w499:dbl, w497:dbl, w498:dbl)
        n171 = property on="Red index" class="DigNum (strict)"("Value"=w498) -> ()  [unwired: 2 in, 2 out]
        n172 = property class="DigNum (strict)"(reference=w519, "Value"=w500) -> ()  [unwired: 1 in, 2 out]
        n173 = property class="DigNum (strict)"(reference=w518, error in=w510, "Value"=w499) -> (error out=w509:errorcluster)  [unwired: 1 out]
        n174 = property on="Blue index" class="DigNum (strict)"("Value"=w497) -> ()  [unwired: 2 in, 2 out]
        n175 = control-ref of="This VI"() -> (w507:refnum<vi>)
        n176 = property class="VI"(reference=w507, error in=w509) -> (reference out=w508:refnum<vi>, error out=w503:errorcluster, "Panel"=w506:refnum<vi>)
        n177 = property class="Pnl"(reference=w506, error in=w503, "DeferPanUpdts"=FALSE ("Defer Panel Updates")) -> (error out=w504:errorcluster)  [unwired: 1 out]
        n178 = Close Reference(reference=w508, error in (no error)=w504) -> ()  [unwired: 1 out]
      }
      event User Event {
        n179 = event-data() -> ("Tangentmode"=w549:bool, "Msg"=w548:string)  [unwired: 1 in]
        n180 = case shown="\"Set Tangent Mode\"" w548 {
          tunnel: w551 -> [_ w562]
          tunnel: w550 -> [_ w561]
          tunnel: w549 -> [_ w560]
          frame "", Default {
          }
          frame "Set Tangent Mode" {
            n181 = Build Array(w562, w561) -> (w563:refnum<vi>[])
            n182 = for {
              tunnel: picture data[5B] ("Plot Images:Front") -> [w573]
              tunnel: w563 -> [w572] mode=indexing
              tunnel: w560 -> [w569]
              tunnel: [w567] -> w559 mode=indexing
              tunnel: [w565] -> w552
              n183 = property class="WFGraph (strict)"(reference=w572, "PlotImages.Front"=w573) -> (reference out=w574:refnum<vi>, error out=w571:errorcluster)  [unwired: 1 in]
              n184 = call "SetCursorNamePosition(SubVI).vi"("Graph"=w574) -> ("Graph Out"=w576:refnum<vi>)
              n185 = call "SetCursorMode.vi"("Visible"=w569, "Graph Refnum"=w576) -> ("Graph Refnum 2"=w575:refnum<vi>)  [unwired: 9 in]
              n186 = call "SetCursorNamePosition(SubVI).vi"("Graph"=w575) -> ("Graph Out"=w570:refnum<vi>)
              n187 = case shown="False" w569 {
                selector: w569 -> [w577 w583]
                tunnel: w571 -> [w581 w585]
                tunnel: [w580 w585] -> w566
                tunnel: w570 -> [w579 w584]
                tunnel: [w578 w584] -> w568
                tunnel: [w577 w583] -> w565
                frame False {
                  n188 = property class="WFGraph (strict)"(reference=w579, error in=w581, "ActPaletteTool"=0 ("Palette:Active Tool")) -> (reference out=w578:refnum<vi>, error out=w580:errorcluster)
                }
                frame True {
                }
              }
              n189 = call "Hide Dynamic Tangent.vi"("error in (no error)"=w566, "Residuals"=w565, "WaveformGraph in"=w568) -> ("WaveformGraph out"=w567:refnum<vi>)  [unwired: 7 in, 1 out]
            }
            n190 = Index Array(array=w559) -> (element #1=w558:refnum<vi>, element #2=w557:refnum<vi>)  [unwired: 2 in]
            n191 = call "AE Variables.vi"("Action"=Enum_Variables."Get Red Cursors") -> ("Dbl Array"=w553:dbl[][])  [unwired: 11 in, 7 out]
            n192 = call "AE Variables.vi"("Action"=Enum_Variables."Get Blue Cursors") -> ("Dbl Array"=w555:dbl[][])  [unwired: 11 in, 7 out]
            n193 = call "DrawCursorLinesFromMem.vi"("CursorMode"=w552, "RedPositionArray"=w553, "BluePositionArray"=w555, "Red"=w557, "Blue"=w558) -> ()  [unwired: 7 in]
          }
        }
      }
      event "GraphSelection(Red:F)": Value Change {
        n194 = event-data() -> ()  [unwired: 1 in, 5 out]
      }
      event "System Stop Button": Value Change {
        n195 = event-data() -> ()  [unwired: 1 in, 5 out]
      }
      event "ZoomRedBtn", "ResetRedBtn": Value Change {
        n196 = event-data() -> ()  [unwired: 1 in, 5 out]
        n197 = case shown="True" "ResetRedBtn" {
          tunnel: w593 -> [_ w602]
          tunnel: w594 -> [_ w601]
          frame False {
          }
          frame True {
            n198 = property class="WFGraph (strict)"(reference=w602, "ActPaletteTool"=5 ("Palette:Active Tool")) -> (reference out=w603:refnum<vi>)  [unwired: 1 in, 1 out]
            n199 = property class="WFGraph (strict)"(reference=w603, "ActPaletteTool"=0 ("Palette:Active Tool")) -> ()  [unwired: 1 in, 2 out]
            n200 = Enqueue Element(queue=w601, element=cluster{"Msg":string, "Data":variant} {"Msg"="Update", "Data"=variant}) -> ()  [unwired: 2 in, 3 out]
          }
        }
        n201 = case shown="True" "ZoomRedBtn" {
          tunnel: w593 -> [_ w606]
          frame False {
          }
          frame True {
            n202 = property class="WFGraph (strict)"(reference=w606, "ActPaletteTool"=2 ("Palette:Active Tool")) -> ()  [unwired: 1 in, 2 out]
            n203 = call "AE User Events.vi"("Action"=Enum_User_Events."User Event", "User Event"="TangentMode") -> ()  [unwired: 8 in, 2 out]
          }
        }
      }
      event "ZoomBlueBtn", "ResetBlueBtn": Value Change {
        n204 = event-data() -> ()  [unwired: 1 in, 5 out]
        n205 = case shown="True" "ResetBlueBtn" {
          tunnel: w610 -> [_ w625]
          tunnel: w611 -> [_ w622]
          frame False {
          }
          frame True {
            n206 = property class="WFGraph (strict)"(reference=w625, "ActPaletteTool"=5 ("Palette:Active Tool")) -> (reference out=w623:refnum<vi>)  [unwired: 1 in, 1 out]
            n207 = property class="WFGraph (strict)"(reference=w623, "ActPaletteTool"=0 ("Palette:Active Tool")) -> ()  [unwired: 1 in, 2 out]
            n208 = Enqueue Element(queue=w622, element=cluster{"Msg":string, "Data":variant} {"Msg"="Update", "Data"=variant}) -> ()  [unwired: 2 in, 3 out]
          }
        }
        n209 = case shown="True" "ZoomBlueBtn" {
          tunnel: w610 -> [_ w619]
          frame False {
          }
          frame True {
            n210 = property class="WFGraph (strict)"(reference=w619, "ActPaletteTool"=2 ("Palette:Active Tool")) -> ()  [unwired: 1 in, 2 out]
            n211 = call "AE User Events.vi"("Action"=Enum_User_Events."User Event", "User Event"="TangentMode") -> ()  [unwired: 8 in, 2 out]
          }
        }
      }
      event "Blue": Shortcut Menu Selection (User) {
        n212 = event-data() -> ("CtlRef"=w627:refnum<vi>, "ItemTag"=w630:string)  [unwired: 1 in, 5 out]
        n213 = control-ref of="Red Pressure"() -> (w629:refnum<vi>)
        n214 = control-ref of="Blue Pressure"() -> (w628:refnum<vi>)
        n215 = case shown="\"SaveImagePDF\"" w630 {
          tunnel: w627 -> [_ w634 _ _]
          tunnel: w629 -> [_ _ w636 w644]
          tunnel: w628 -> [_ _ w637 w643]
          frame "False", Default {
          }
          frame "ZoomOut" {
            n216 = property class="WFGraph (strict)"(reference=w634, "ActPaletteTool"=5 ("Palette:Active Tool")) -> ()  [unwired: 1 in, 2 out]
          }
          frame "SaveImagePDF" {
            n217 = property class="DigNum (strict)"(reference=w636) -> ("Value"=w638:dbl)  [unwired: 1 in, 2 out]
            n218 = property class="DigNum (strict)"(reference=w637) -> ("Value"=w639:dbl)  [unwired: 1 in, 2 out]
            n219 = control-ref of="Blue"() -> (w641:refnum<vi>)
            n220 = control-ref of="Red"() -> (w640:refnum<vi>)
            n221 = call-by-ref "?"("RedPressure"=w638, "BluePressure"=w639, "Print"=FALSE, "Blue Graph Refnum"=w641, "Red Graph Refnum"=w640) -> ()  [unwired: 7 in, 2 out]
          }
          frame "PrintImages" {
            n222 = property class="DigNum (strict)"(reference=w644) -> ("Value"=w646:dbl)  [unwired: 1 in, 2 out]
            n223 = property class="DigNum (strict)"(reference=w643) -> ("Value"=w645:dbl)  [unwired: 1 in, 2 out]
            n224 = control-ref of="Blue"() -> (w648:refnum<vi>)
            n225 = control-ref of="Red"() -> (w647:refnum<vi>)
            n226 = call-by-ref "?"("RedPressure"=w646, "BluePressure"=w645, "Print"=TRUE, "Blue Graph Refnum"=w648, "Red Graph Refnum"=w647) -> ()  [unwired: 7 in, 2 out]
          }
        }
      }
      event "Red": Shortcut Menu Selection (User) {
        n227 = event-data() -> ("CtlRef"=w650:refnum<vi>, "ItemTag"=w653:string)  [unwired: 1 in, 5 out]
        n228 = control-ref of="Blue Pressure"() -> (w651:refnum<vi>)
        n229 = control-ref of="Red Pressure"() -> (w652:refnum<vi>)
        n230 = case shown="\"SaveImagePDF\"" w653 {
          tunnel: w650 -> [_ w657 _ _]
          tunnel: w652 -> [_ _ w660 w666]
          tunnel: w651 -> [_ _ w659 w667]
          frame "False", Default {
          }
          frame "ZoomOut" {
            n231 = property class="WFGraph (strict)"(reference=w657, "ActPaletteTool"=5 ("Palette:Active Tool")) -> ()  [unwired: 1 in, 2 out]
          }
          frame "SaveImagePDF" {
            n232 = property class="DigNum (strict)"(reference=w660) -> ("Value"=w661:dbl)  [unwired: 1 in, 2 out]
            n233 = property class="DigNum (strict)"(reference=w659) -> ("Value"=w662:dbl)  [unwired: 1 in, 2 out]
            n234 = control-ref of="Blue"() -> (w664:refnum<vi>)
            n235 = control-ref of="Red"() -> (w663:refnum<vi>)
            n236 = call-by-ref "?"("RedPressure"=w661, "BluePressure"=w662, "Print"=FALSE, "Blue Graph Refnum"=w664, "Red Graph Refnum"=w663) -> ()  [unwired: 7 in, 2 out]
          }
          frame "PrintImages" {
            n237 = property class="DigNum (strict)"(reference=w666) -> ("Value"=w669:dbl)  [unwired: 1 in, 2 out]
            n238 = property class="DigNum (strict)"(reference=w667) -> ("Value"=w668:dbl)  [unwired: 1 in, 2 out]
            n239 = control-ref of="Blue"() -> (w671:refnum<vi>)
            n240 = control-ref of="Red"() -> (w670:refnum<vi>)
            n241 = call-by-ref "?"("RedPressure"=w669, "BluePressure"=w668, "Print"=TRUE, "Blue Graph Refnum"=w671, "Red Graph Refnum"=w670) -> ()  [unwired: 7 in, 2 out]
          }
        }
      }
      event "Red", "Blue": Shortcut Menu Activation? {
        n242 = event-data() -> ("MenuRef"=w682:refnum<k9>)  [unwired: 1 in]
        n243 = call "AE Variables.vi"("Action"=Enum_Variables."Get Language") -> ("RingOut"=w676:u16)  [unwired: 11 in, 7 out]
        n244 = Delete Menu Items(9:w682) -> (0:w680:errorcluster, 3:w681:refnum<k9>)  [unwired: 3 in]
        n245 = case shown="0, Default" w676 {
          tunnel: [string[] ["Zoom Ud", "Gem Grafer i PDF", "Print Grafer"] ("item names") string[] ["Zoom Out", "Save Graphs as PDF", "Print Graphs"] ("item names") string[] ["Zoom Out", "Save Graphs as PDF", "Print Graphs"] ("item names")] -> w679
          frame 0, Default {
          }
          frame 1 {
          }
          frame 2 {
          }
        }
        n246 = Insert Menu Items(6:w680, 7:string[] ["ZoomOut", "SaveImagePDF", "PrintImages"] ("item tags"), 8:w679, 9:w681) -> ()  [unwired: 2 in, 3 out]
        n247 = event-data() -> ()  [unwired: 2 in, 1 out]
      }
      event Pane Size {
        n248 = event-data() -> ()  [unwired: 1 in, 1 out]
        n249 = Enqueue Element(queue=w690, element=cluster{"Msg":string, "Data":variant} {"Msg"="Update", "Data"=variant}) -> ()  [unwired: 2 in, 3 out]
      }
    }
  }
  n250 = call <vilib>:"General Error Handler.vi"("error in (no error)"=w7) -> ()  [unwired: 10 in, 5 out]
  n251 = Destroy User Event(user event=w6, error in=w7) -> (error out=w8:errorcluster)
  n252 = Unregister For Events(event registration refnum=w9, error in=w8) -> (error out=w5:errorcluster)
  n253 = Release Queue(queue="Queue", force destroy? (F)=TRUE, error in (no error)=w12) -> ()  [unwired: 3 out]
  n254 = call <vilib>:"Clear Errors.vi"("error in (no error)"=w5) -> ()  [unwired: 6 in, 1 out]
